vi "Format Client Request (String).vi"(8 "error in (no error)":errorcluster, 9 "id":string, 10 "params":refnum<class "JSON Object.lvclass">, 11 "method":string) -> (0 "error out":errorcluster, 2 "Request String":string)   [LabVIEW 2016, in "JSONRPC Server.lvclass"]
uses:
  JSONRPC Server.lvclass
  <vilib>/NI/JSON Support for LabVIEW/JSON Data Classes/JSON Object/JSON Object.lvclass
  C:/Program Files (x86)/National Instruments/LabVIEW 2016/vi.lib/NI/JSON Support for LabVIEW/JSON Data Classes/JSON Datatype/JSON Null.lvclass
  <vilib>/NI/JSON Support for LabVIEW/JSON Data Classes/JSON Object/Insert Key Value Pair (Single String).vi
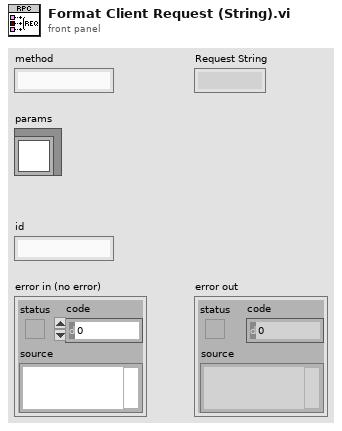
[diagram p1: front panel]
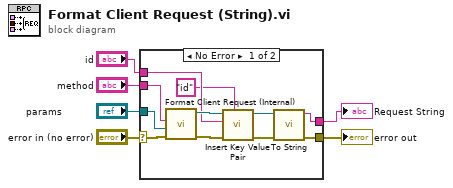
[diagram p0: block diagram]
diagram:
  n1 = case shown="No Error" "error in (no error)" {
    selector: "error in (no error)" -> [w17 w18]
    tunnel: [w16 w18] -> w5
    tunnel: "params" -> [w11 _]
    tunnel: [w15 _] -> w3
    tunnel: "method" -> [w14 _]
    tunnel: "id" -> [w9 _]
    frame No Error {
      n2 = call "Format Client Request (Internal).vi"("error in (no error)"=w17, "params"=w11, "method"=w14) -> ("error out"=w12:errorcluster, "JSON Object out"=w10:refnum<class "JSON Object.lvclass">)  [unwired: 7 in]
      n3 = call-poly <vilib>:"Insert Key Value Pair.vi"("key"="id" ("Name"), "error in (no error)"=w12, "value"=w9, "JSON Object in"=w10) -> ("error out"=w13:errorcluster, "JSON Object out"=w7:refnum<class "JSON Object.lvclass">)  [unwired: 5 in, 1 out]
      n4 = call-dynamic "To String.vi"("error in (no error)"=w13, "JSON Object in"=w7) -> ("error out"=w16:errorcluster, "String"=w15:string)  [unwired: 8 in]
    }
    frame Error {
    }
  }
  "error out" <- w5
  "Request String" <- w3
